vi "Check if Open or Locked.vi"(8 "error in (no error)":errorcluster, 11 "Missing VI Type in":refnum<class "Missing VI Type.lvclass">) -> (0 "error out":errorcluster, 3 "Openable?":bool)   [LabVIEW 2020, in "Peek Window.lvlib" / "Missing VI Type.lvclass"]
uses:
  Missing VI Type.lvclass
  Missing VI Type.lvclass/Missing VI Type.ctl
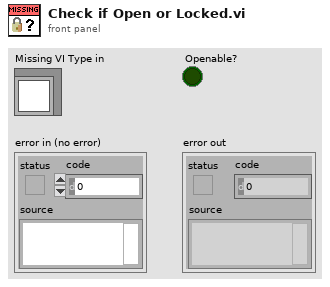
[diagram p1: front panel]
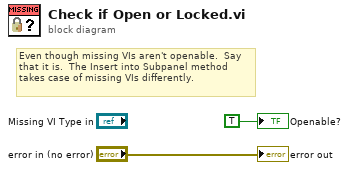
[diagram p0: block diagram]
diagram:
  # "Even though missing VIs aren't openable.  Say that it is.  The Insert into Subpanel method takes case of missing VIs differently."
  "error out" <- "error in (no error)"
  "Openable?" <- TRUE
